vi "Auto Position Drive.vi"(9 "Desired Position":dbl, 11 "Current Position":dbl) -> (2 "Finished?":bool)   [LabVIEW 2015]
uses:
  Common Code/Drivetrain Modes.ctl
  Robot Global Data.vi
panel:
  out "Position":i8
  # "Position #1 = Low bar\nPosition #2 = what ever next to lowbar\netc."
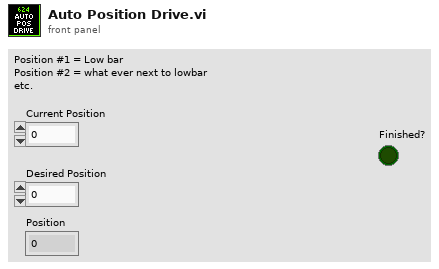
[diagram p1: front panel]
types:
  T1 = typedef "Drivetrain Modes.ctl" = enum16{"Tank", "Climb", "Manual", "Goal Vision Targeting", "PID Distance Drive", "Hybrid", "Gyro Steer"}
  T2 = typedef "Drivetrain Status Cluster.ctl" = cluster{"Modes":T1, "Y (Throttle)":dbl, "X (Steer)":dbl, "Gyro In Range?":bool, "Distance Drive Finished?":bool, "Stop Eject Lockout":bool, "Dist Drive Status":T3, "Y Target":dbl, "Heading Target":dbl, "Vision Target Aligned?":bool, "Gear":dbl, "1st Gear Time":dbl, "2nd Gear Time":dbl, "1st Gear Shifts":dbl, "2nd Gear Shifts":dbl}
  T3 = typedef "Dist Drive Status.ctl" = cluster{"Y In Range":bool, "X In Range":bool, "Gyro In Range":bool, "Y Dist":dbl, "X Dist":dbl, "Gyro":dbl}
  T4 = typedef "Drivetrain Commands.ctl" = cluster{"Y Power":dbl, "Turn Power":dbl, "1st Gear?":bool, "Modes":T1, "Heading Target":dbl, "X Max Speed":dbl, "Y Max Speed":dbl, "X Min Speed":dbl, "Y Min Speed":dbl, "Y Target":dbl, "Max Accel":dbl, "Max Velocity":dbl, "Y Power 2":dbl, "Pivot Speed":dbl}
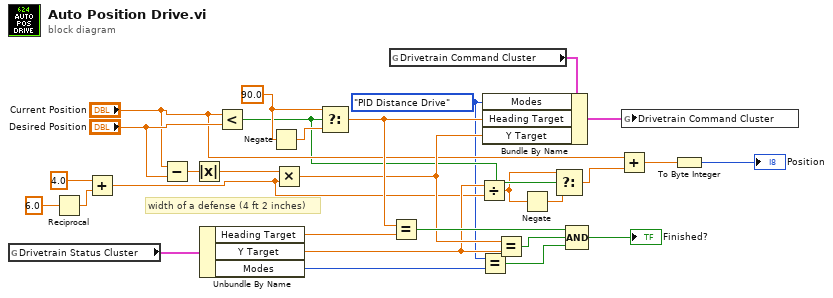
[diagram p0: block diagram]
diagram:
  w3 = Drivetrain_Modes."PID Distance Drive" ("Modes")
  w28 = 90.0
  # "width of a defense (4 ft 2 inches)"
  n1 = global read "Robot Global Data.vi" "Drivetrain Status Cluster"() -> (w25:T2)
  n2 = Reciprocal(x=6.0) -> (1/x=w8:dbl)
  n3 = Add(x=4.0, y=w8) -> (x+y=w6:dbl)
  n4 = Subtract(x="Current Position", y="Desired Position") -> (x-y=w19:dbl)
  n5 = Absolute Value(x=w19) -> (abs(x)=w18:dbl)
  n6 = Unbundle By Name(w25) -> ("Heading Target"=w23:dbl, "Y Target"=w13:dbl, "Modes"=w2:T1)
  n7 = Less?(x="Current Position", y="Desired Position") -> (x < y?=w12:bool)
  n8 = Negate(x=w28) -> (-x=w29:dbl)
  n9 = Multiply(x=w18, y=w6) -> (x*y=w17:dbl)
  n10 = Select(t=w28, s=w12, f=w29) -> (s? t:f=w24:dbl)
  n11 = global read "Robot Global Data.vi" "Drivetrain Command Cluster"() -> (w27:T4)
  n12 = Equal?(x=w24, y=w23) -> (x = y?=w22:bool)
  n13 = Divide(x=w13, y=w6) -> (x/y=w11:dbl)
  n14 = Equal?(x=w3, y=w2) -> (x = y?=w1:bool)
  n15 = Bundle By Name(cluster=w27, "Modes"=w3, "Heading Target"=w24, "Y Target"=w17) -> (w26:T4)
  n16 = Equal?(x=w17, y=w13) -> (x = y?=w16:bool)
  n17 = Negate(x=w11) -> (-x=w10:dbl)
  n18 = Select(t=w11, s=w12, f=w10) -> (s? t:f=w14:dbl)
  n19 = Compound Arithmetic op=AND(w22, w16, w1) -> (→"Finished?":bool)
  n20 = Add(x="Current Position", y=w14) -> (x+y=w5:dbl)
  n21 = global write "Robot Global Data.vi" "Drivetrain Command Cluster"(w26) -> ()
  n22 = To Byte Integer(number=w5) -> (8bit integer=→"Position":i8)
